vi "Readout.vi"(8 "Error In":errorcluster, 11 "BNT_ULx-MCSV in":refnum<class "BNT_ULx-MCSV.lvclass">) -> (0 "Error Out":errorcluster, 2 "CSPP_DataCollection out":refnum<class "CSPP_DataCollection.lvclass">, 3 "BNT_ULx-MCSV out":refnum<class "BNT_ULx-MCSV.lvclass">)   [LabVIEW 2020, in "BNT_ULx.lvlib" / "BNT_ULx-MCSV.lvclass"]
doc: "Read single value from multiple channels."
uses:
  BNT_ULx-MCSV.lvclass
  CSPP_Core/Classes/CSPP_BaseClasses/DataCollection/CSPP_DataCollection.lvclass
  C:/User/Brand/LVP/CSPP/CSPP-Template/Packages/CSPP_Core/Actors/CSPP_BaseActor/CSPP_BaseActor.lvclass
  C:/Program Files (x86)/National Instruments/LabVIEW 2020/vi.lib/ActorFramework/Actor/Actor.lvclass
  CSPP_Core/Messages/CSPP_DataUpdate Msg/CSPP_DataUpdate Msg.lvclass
  BNT_ULx-MCSV-Data/BNT_ULx-MCSV-Data.lvclass
  C:/User/Brand/LVP/CSPP/CSPP-Template/Packages/CSPP_Core/Classes/CSPP_BaseClasses/Data/CSPP_Data.lvclass
  BNT_ULx-MCSV.lvclass/BNT_ULx-MCSV.ctl
  CSPP_Core/Actors/CSPP_BaseActor/CSPP_BaseActor.lvclass/CSPP_BaseActor.ctl
  CSPP_Core/Classes/CSPP_BaseClasses/Data/CSPP_Data.lvclass/CSPP_Data.ctl
  CSPP_Core/Classes/CSPP_BaseClasses/DataCollection/CSPP_DataCollection.lvclass/CSPP_DataCollection.ctl
  <vilib>/ActorFramework/Actor/Actor.lvclass/Actor.ctl
  <vilib>/ActorFramework/Message Enqueuer/Message Enqueuer.lvclass/Message Enqueuer.ctl
  CSPP_Core/Classes/CSPP_BaseClasses/Data/Write Error.vi
  CSPP_Core/Classes/CSPP_BaseClasses/Data/Write Time Stamp.vi
  <vilib>/ActorFramework/Message Enqueuer/Init from Existing Queue.vi
  <vilib>/ULx/Read.llb/ULx Read (Counter 1D DBL NChan 1Samp).vi
  <vilib>/ULx/Read.llb/ULx Read (Digital 1D Bool NChan 1Samp 1Line).vi
  <vilib>/ActorFramework/Message Enqueuer/Message Enqueuer.lvclass
  CSPP_Core/Actors/CSPP_BaseActor/CSPP_BaseActor.lvclass
  <vilib>/ActorFramework/Actor/Actor.lvclass
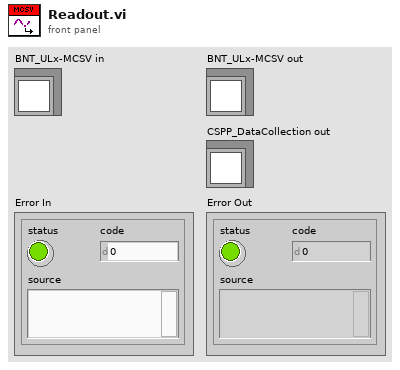
[diagram p1: front panel]
types:
  T1 = cluster{"CSPP_DataUpdate Msg":refnum<class "CSPP_DataUpdate Msg.lvclass">, "Receiver":refnum<class "Message Enqueuer.lvclass">}
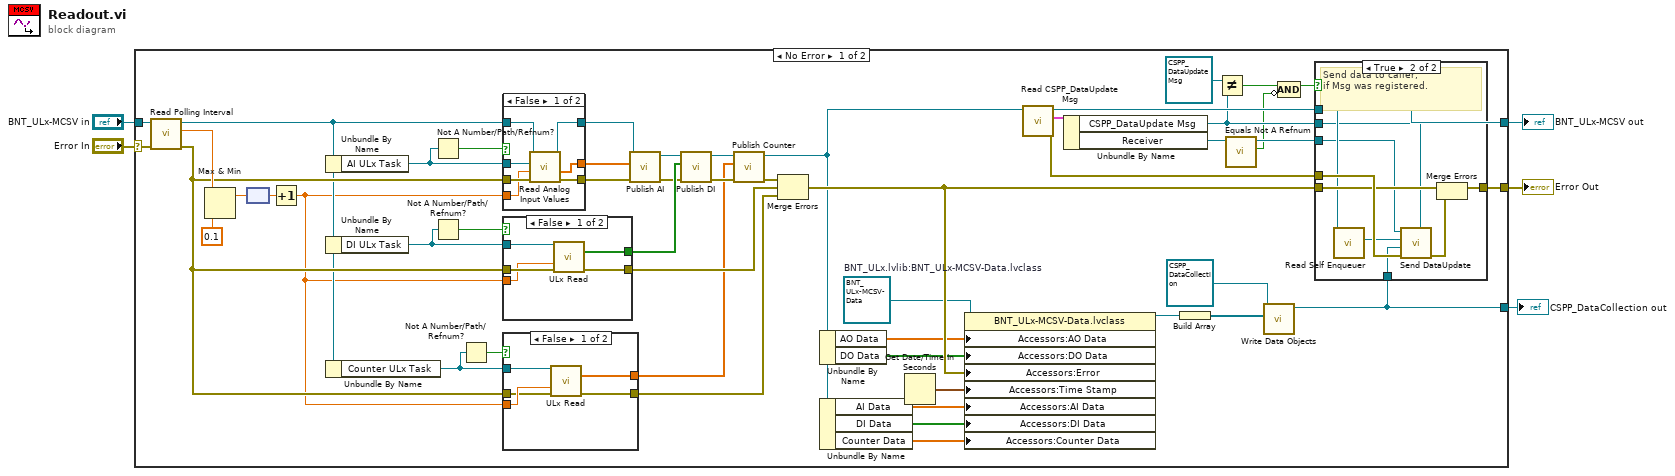
[diagram p0: block diagram]
diagram:
  n1 = case shown="No Error" "Error In" {
    selector: "Error In" -> [w54 w88]
    tunnel: [w42 w88] -> w4
    tunnel: [w25 w87] -> w2
    tunnel: "BNT_ULx-MCSV in" -> [w55 w87]
    tunnel: [w30 _] -> w1
    frame No Error {
      w6 = refnum<class "BNT_ULx-MCSV-Data.lvclass"> refnum  # BNT_ULx.lvlib:BNT_ULx-MCSV-Data.lvclass
      n2 = call "Read Polling Interval.vi"("error in (no error)"=w54, "CSPP_BaseActor in"=w55) -> ("error out"=w41:errorcluster, "Polling Interval"=w53:dbl[unit], "CSPP_BaseActor out"=w28:refnum<class "BNT_ULx-MCSV.lvclass">)  [unwired: 7 in]
      n3 = Max & Min(x=w53, y=dbl[unit] 0.1) -> (max(x,y)=w51:dbl[unit])  [unwired: 1 out]
      n4 = node(w51) -> (w44:dbl)
      n5 = Increment(x=w44) -> (x+1=w26:dbl)
      n6 = Unbundle By Name(w28) -> ("AI ULx Task"=w27:refnum<k24>)
      n7 = Unbundle By Name(w28) -> ("DI ULx Task"=w48:refnum<k24>)
      n8 = Unbundle By Name(w28) -> ("Counter ULx Task"=w45:refnum<k24>)
      n9 = Not A Number/Path/Refnum?(number/path/refnum=w27) -> (NaN/Path/Refnum?=w49:bool)
      n10 = Not A Number/Path/Refnum?(number/path/refnum=w48) -> (NaN/Path/Refnum?=w47:bool)
      n11 = Not A Number/Path/Refnum?(number/path/refnum=w45) -> (NaN/Path/Refnum?=w46:bool)
      n12 = case shown="False" w49 {
        tunnel: [w63 w70] -> w22
        tunnel: w26 -> [w66 _]
        tunnel: w41 -> [w67 w70]
        tunnel: w28 -> [w68 w69]
        tunnel: [w64 w69] -> w23
        tunnel: w27 -> [w65 _]
        tunnel: [w62 _] -> w21
        frame False {
          n13 = call-dynamic "Read Analog Input Values.vi"("error in"=w67, "Timeout / s"=w66, "AI ULx Task"=w65, "BNT_ULx-MCSV in"=w68) -> ("error out"=w63:errorcluster, "AI Data"=w62:dbl[], "BNT_ULx-MCSV out"=w64:refnum<class "BNT_ULx-MCSV.lvclass">)  [unwired: 5 in]
        }
        frame True {
        }
      }
      n14 = case shown="False" w47 {
        tunnel: w48 -> [w60 _]
        tunnel: w26 -> [w57 _]
        tunnel: [w56 _] -> w19
        tunnel: [w59 w61] -> w50
        tunnel: w41 -> [w58 w61]
        frame False {
          n15 = call-poly <vilib>:"ULx Read.vi"("task in"=w60, "timeout"=w57, "error in"=w58) -> ("data"=w56:bool[], "error out"=w59:errorcluster)  [unwired: 10 in, 1 out]
        }
        frame True {
        }
      }
      n16 = case shown="False" w46 {
        tunnel: w45 -> [w74 _]
        tunnel: w26 -> [w73 _]
        tunnel: [w71 _] -> w13
        tunnel: [w75 w76] -> w43
        tunnel: w41 -> [w72 w76]
        frame False {
          n17 = call-poly <vilib>:"ULx Read.vi"("task in"=w74, "timeout"=w73, "error in"=w72) -> ("data"=w71:dbl[], "error out"=w75:errorcluster)  [unwired: 10 in, 1 out]
        }
        frame True {
        }
      }
      n18 = call "Publish AI.vi"("error in"=w22, "AI Data"=w21, "BNT_ULx-MCSV in"=w23) -> ("error out"=w18:errorcluster, "BNT_ULx-MCSV out"=w17:refnum<class "BNT_ULx-MCSV.lvclass">)  [unwired: 7 in]
      n19 = call "Publish DI.vi"("error in"=w18, "DI Data"=w19, "BNT_ULx-MCSV in"=w17) -> ("error out"=w15:errorcluster, "BNT_ULx-MCSV out"=w16:refnum<class "BNT_ULx-MCSV.lvclass">)  [unwired: 7 in]
      n20 = call "Publish Counter.vi"("error in"=w15, "Counter Data"=w13, "BNT_ULx-MCSV in"=w16) -> ("error out"=w14:errorcluster, "BNT_ULx-MCSV out"=w11:refnum<class "BNT_ULx-MCSV.lvclass">)  [unwired: 7 in]
      n21 = Merge Errors(w14, w50, w43) -> (w39:errorcluster)
      n22 = Unbundle By Name(w11) -> ("AO Data"=w35:dbl[], "DO Data"=w34:bool[])
      n23 = Unbundle By Name(w11) -> ("AI Data"=w24:dbl[], "DI Data"=w20:bool[], "Counter Data"=w12:dbl[])
      n24 = Get Date/Time In Seconds() -> (seconds since 1Jan1904=w36:timestamp)
      n25 = property class="BNT_ULx-MCSV-Data.lvclass"(reference=w6, "Accessors:AO Data"=w35, "Accessors:DO Data"=w34, "Accessors:Error"=w39, "Accessors:Time Stamp"=w36, "Accessors:AI Data"=w24, "Accessors:DI Data"=w20, "Accessors:Counter Data"=w12) -> (reference out=w32:refnum<class "BNT_ULx-MCSV-Data.lvclass">)  [unwired: 1 in, 1 out]
      n26 = call-dynamic "Read CSPP_DataUpdate Msg.vi"("CSPP_BaseActor in"=w11) -> ("error out"=w40:errorcluster, "CSPP_DataUpdate Msg"=w38:T1, "CSPP_BaseActor out"=w25:refnum<class "BNT_ULx-MCSV.lvclass">)  [unwired: 8 in]
      n27 = Unbundle By Name(w38) -> ("CSPP_DataUpdate Msg"=w10:refnum<class "CSPP_DataUpdate Msg.lvclass">, "Receiver"=w9:refnum<class "Message Enqueuer.lvclass">)
      n28 = Build Array(w32) -> (w31:refnum<class "BNT_ULx-MCSV-Data.lvclass">[])
      n29 = Not Equal?(x=refnum<class "CSPP_DataUpdate Msg.lvclass"> refnum ("CSPP_DataUpdate Msg.lvclass"), y=w10) -> (x != y?=w29:bool)
      n30 = call <vilib>:"Equals Not A Refnum.vi"("Message Enqueuer"=w9) -> ("Not a refnum?"=w7:bool)  [unwired: 10 in]
      n31 = call "Write Data Objects.vi"("Data Objects"=w31, "CSPP_DataCollection in"=refnum<class "CSPP_DataCollection.lvclass"> refnum ("CSPP_BaseClasses.lvlib:CSPP_DataCollection.lvclass")) -> ("CSPP_DataCollection out"=w30:refnum<class "CSPP_DataCollection.lvclass">)  [unwired: 8 in, 1 out]
      n32 = Compound Arithmetic op=AND(w29, invert w7) -> (w8:bool)
      n33 = case shown="True" w8 {
        tunnel: [w77 w86] -> w42
        tunnel: w40 -> [_ w85]
        tunnel: w39 -> [w77 w84]
        tunnel: w25 -> [_ w83]
        tunnel: w30 -> [_ w80]
        tunnel: w10 -> [_ w79]
        tunnel: w9 -> [_ w78]
        frame False {
        }
        frame True {
          # "Send data to caller, \nif Msg was registered."
          n34 = call <vilib>:"Read Self Enqueuer.vi"("Actor"=w83) -> ("Self Enqueuer"=w82:refnum<class "Message Enqueuer.lvclass">)  [unwired: 10 in]
          n35 = call "Send DataUpdate.vi"("CSPP_DataUpdate Msg"=w79, "error in (no error)"=w85, "CSPP_DataCollection"=w80, "Sender Enqueuer"=w82, "Message Enqueuer"=w78) -> ("error out"=w81:errorcluster)  [unwired: 5 in, 1 out]
          n36 = Merge Errors(w84, w81) -> (w86:errorcluster)
        }
      }
    }
    frame Error {
    }
  }
  "Error Out" <- w4
  "BNT_ULx-MCSV out" <- w2
  "CSPP_DataCollection out" <- w1
